vi "Add Resource (Rx DSP).vi"(0 "acq in":refnum<class "niUSRP Rx DSP v2 FPGA.lvclass">, 1 "instance (0)":u8) -> (4 "output cluster":refnum<class "niUSRP Rx DSP v2 FPGA.lvclass">)   [LabVIEW 2025, in "niUSRP Rx DSP v2 FPGA.lvclass"]
uses:
  niUSRP Rx DSP v2 FPGA.lvclass
  Public/Typedefs/DSP Shared Regs.ctl
  niUSRP Rx DSP v2 FPGA.lvclass/niUSRP Rx DSP v2 FPGA.ctl
  <vilib>/rvi/DataTransferAndStorage/Container/Common/niFpgaContainerGetUniqueNameForEmu.vi
  <vilib>/rvi/DataTransferAndStorage/Container/Common/niFpgaContainerSetEmuInfo.vi
  <vilib>/rvi/eio/common/nirviEmuReportErrorAndStop.vi
  <vilib>/rvi/LocalResourceManager/LocalResourceManager.xnode
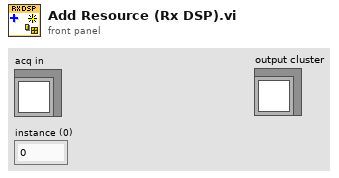
[diagram p1: front panel]
types:
  T1 = typedef "niUSRP Rx DSP v2 FPGA.lvclass/DSP Shared Regs.ctl" = cluster{"rfsa.abort":refnum<k21>, "reset":refnum<k21>, "reset.done":refnum<k21>, "RxDspEnabled":refnum<k21>}
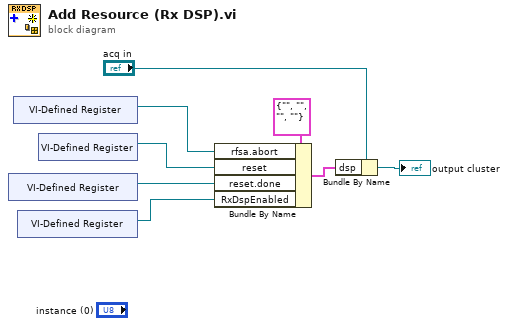
[diagram p0: block diagram]
diagram:
  n1 = xnode "VI-Defined Register"() -> ("Register Out"=w7:refnum<k21>)
  n2 = xnode "VI-Defined Register"() -> ("Register Out"=w6:refnum<k21>)
  n3 = xnode "VI-Defined Register"() -> ("Register Out"=w1:refnum<k21>)
  n4 = xnode "VI-Defined Register"() -> ("Register Out"=w8:refnum<k21>)
  n5 = Bundle By Name(cluster=T1 {"rfsa.abort"="", "reset"="", "reset.done"="", "RxDspEnabled"=""} ("dsp"), "rfsa.abort"=w6, "reset"=w8, "reset.done"=w7, "RxDspEnabled"=w1) -> (w2:T1)
  n6 = Bundle By Name(cluster="acq in", "dsp"=w2) -> (→"output cluster":refnum<class "niUSRP Rx DSP v2 FPGA.lvclass">)
